vi "Read Unified Leaf.vi"(11 "Base Attributes in":refnum<class "Base Attributes.lvclass">) -> (2 "Unified Leaf":bool)   [LabVIEW 2020, in "jettl.lvlib" / "Base Attributes.lvlib" / "Base Attributes.lvclass"]
uses:
  Base Attributes.lvclass
  Base Attributes.lvclass/Base Attributes.ctl
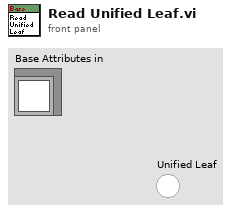
[diagram p1: front panel]
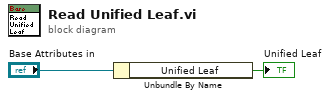
[diagram p0: block diagram]
diagram:
  n1 = Unbundle By Name("Base Attributes in") -> ("Unified Leaf"=→"Unified Leaf":bool)
